vi "OAT Compute Timebase Plot Data.vi"(6 "trigger pulse direction":u16(ring)=1 items=["positive going", "negative going"], 7 "tach duty":i32=1, 8 "actual samples/rev":dbl format="%.2f", 9 "revolutions":dbl format="%.2f", 10 "start":dbl format="%.2f", 11 "timebase plot in":cluster{"X":dbl[], "Y":dbl[]}[](array[cluster]) {"Y" format="%.2f"; "X" format="%.2f"}) -> (2 "Y axis out":cluster{dbl[], dbl[]}[](array[cluster]) {"?" format="%.2f"; "?" format="%.2f"}, 3 "X axis out":cluster{dbl[], dbl[]}[](array[cluster]) {"?" format="%.2f"; "?" format="%.2f"})   [LabVIEW 2017]
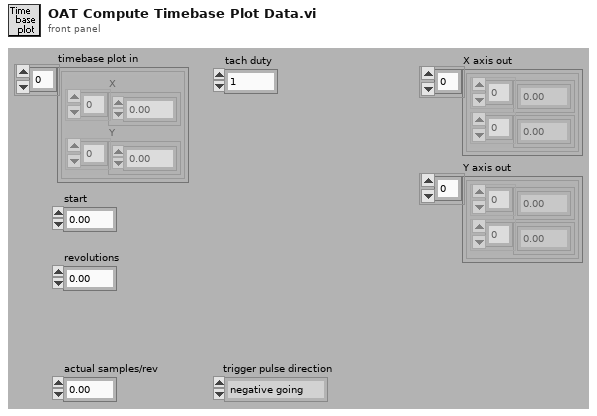
[diagram p1: front panel]
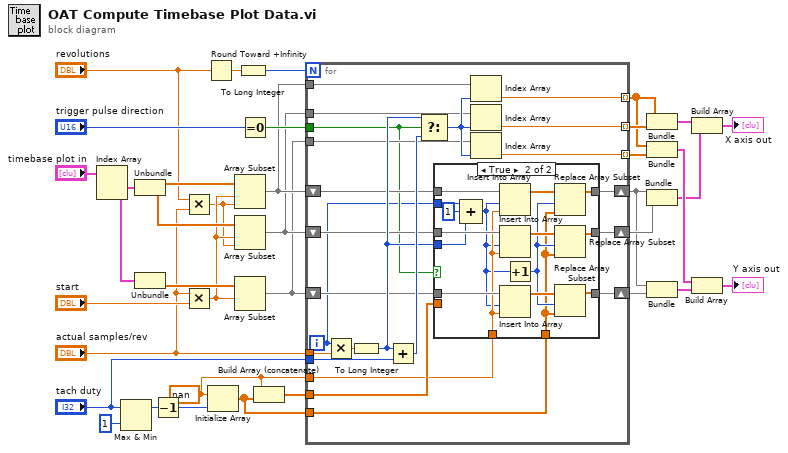
[diagram p0: block diagram]
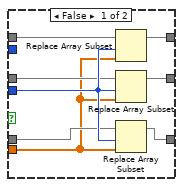
[diagram p2: hidden frame]
diagram:
  w2 = nan ("element")
  n1 = Index Array(array="timebase plot in") -> (element #1=w24:cluster{"X":dbl[], "Y":dbl[]}, element #2=w23:cluster{"X":dbl[], "Y":dbl[]})  [unwired: 2 in]
  n2 = Max & Min(x="tach duty", y=1) -> (max(x,y)=w14:i32)  [unwired: 1 out]
  n3 = Unbundle(w24) -> ("X"=w22:dbl[], "Y"=w21:dbl[])
  n4 = Unbundle(w23) -> ("Y"=w20:dbl[])  [unwired: 1 out]
  n5 = Decrement(x=w14) -> (x-1=w4:i32)
  n6 = Multiply(x="revolutions", y="actual samples/rev") -> (x*y=w15:dbl)
  n7 = Multiply(x="actual samples/rev", y="start") -> (x*y=w19:dbl)
  n8 = Round Toward +Infinity(x="revolutions") -> (ceil(x): smallest int >= x=w34:dbl)
  n9 = Initialize Array(w2, w4) -> (w1:dbl[])
  n10 = Array Subset(array=w22, index=w19, length=w15) -> (w7:dbl[])
  n11 = Array Subset(array=w21, index=w19, length=w15) -> (w6:dbl[])
  n12 = Array Subset(array=w20, index=w19) -> (w5:dbl[])  [unwired: 1 in]
  n13 = To Long Integer(number=w34) -> (32bit integer=w35:i32)
  n14 = Equal To 0?(x="trigger pulse direction") -> (x = 0?=w25:bool)
  n15 = Build Array (concatenate)(w2, w1) -> (w3:dbl[])
  n16 = for {
    N: w35 -> [_]
    tunnel: "actual samples/rev" -> [w54]
    tunnel: [w57] -> w29 mode=indexing
    tunnel: [w56] -> w33 mode=indexing
    tunnel: [w55] -> w30 mode=indexing
    tunnel: w25 -> [w41]
    tunnel: "tach duty" -> [w53]
    shift-right: [w50] -> w11
    shift-left: w7 -> [w51]
    shift-right: [w48] -> w12
    shift-left: w6 -> [w45]
    shift-right: [w49] -> w10
    shift-left: w5 -> [w43]
    tunnel: w7 -> [w47]
    tunnel: w6 -> [w46]
    tunnel: w5 -> [w44]
    tunnel: w3 -> [w42]
    tunnel: w2 -> [w39]
    tunnel: w1 -> [w38]
    i -> [w40]
    n17 = Multiply(x=w40, y=w54) -> (x*y=w60:dbl)
    n18 = To Long Integer(number=w60) -> (32bit integer=w52:i32)
    n19 = Add(x=w52, y=w53) -> (x+y=w59:i32)
    n20 = Select(t=w52, s=w41, f=w59) -> (s? t:f=w58:i32)
    n21 = case shown="True" w41 {
      tunnel: w52 -> [w68 w70]
      tunnel: w51 -> [w67 w84]
      tunnel: [w66 w74] -> w50
      tunnel: [w65 w72] -> w49
      tunnel: [w64 w73] -> w48
      tunnel: w45 -> [w63 w83]
      tunnel: w43 -> [w62 w82]
      tunnel: w42 -> [w61 _]
      tunnel: w40 -> [_ w71]
      tunnel: w39 -> [_ w81]
      tunnel: w38 -> [_ w75]
      frame False {
        n22 = Replace Array Subset(array=w67, new element=w61, index=w68) -> (w66:dbl[])
        n23 = Replace Array Subset(array=w63, new element=w61, index=w68) -> (w64:dbl[])
        n24 = Replace Array Subset(array=w62, new element=w61, index=w68) -> (w65:dbl[])
      }
      frame True {
        n25 = Compound Arithmetic op=ADD(w71, 1 ("value"), w70) -> (w77:i32)
        n26 = Insert Into Array(array=w84, index=w77, new element=w81) -> (w80:dbl[])
        n27 = Insert Into Array(array=w83, index=w77, new element=w81) -> (w79:dbl[])
        n28 = Insert Into Array(array=w82, index=w77, new element=w81) -> (w78:dbl[])
        n29 = Increment(x=w77) -> (x+1=w76:i32)
        n30 = Replace Array Subset(array=w80, new element=w75, index=w76) -> (w74:dbl[])
        n31 = Replace Array Subset(array=w79, new element=w75, index=w76) -> (w73:dbl[])
        n32 = Replace Array Subset(array=w78, new element=w75, index=w76) -> (w72:dbl[])
      }
    }
    n33 = Index Array(array=w47, index=w58) -> (element=w57:dbl)
    n34 = Index Array(array=w46, index=w58) -> (element=w56:dbl)
    n35 = Index Array(array=w44, index=w58) -> (element=w55:dbl)
  }
  n36 = Bundle(w29, w33) -> (w32:cluster{dbl[], dbl[]})  [unwired: 1 in]
  n37 = Bundle(w29, w30) -> (w28:cluster{dbl[], dbl[]})  [unwired: 1 in]
  n38 = Bundle(w11, w12) -> (w9:cluster{dbl[], dbl[]})  [unwired: 1 in]
  n39 = Bundle(w11, w10) -> (w8:cluster{dbl[], dbl[]})  [unwired: 1 in]
  n40 = Build Array(w32, w9) -> (→"X axis out":cluster{dbl[], dbl[]}[])
  n41 = Build Array(w28, w8) -> (→"Y axis out":cluster{dbl[], dbl[]}[])
